vi "configuration UI.vi"() -> ()   [LabVIEW 2013, in "Shared Library Module editor node.lvclass"]
doc: "Platypus Framework 1.0.1.60\nNI Systems Engineering - National Instruments"
uses:
  Shared Library Module editor node.lvclass
  <vilib>/CEF_TreeControl/Node/NodeRef.ctl
  <vilib>/CEF_TreeControl/Node/NISE_CEF_Node.lvclass
  <vilib>/NI/AMC/Message Queue.ctl
  <vilib>/NI/AMC/Message.ctl
  <vilib>/NI/Tools/Keyed Array/KeyedArray.ctl
  <vilib>/CEF_TreeControl/Node/UserEventRef.ctl
  <vilib>/CEF_TreeControl/Controls/EventCluster.ctl
  <vilib>/TBM Modules/CLFN/configuration/Shared Library Module configuration.lvclass
  <vilib>/NI/Module Execution Interface/Engine Configuration/engine configuration.lvclass
  <vilib>/NI/Tag Bus Data Framework/Configuration Editor/Classes/Engine Parent/Engine Parent Editor Node.lvclass
  <vilib>/NI/Tag Bus Module Framework/root configuration/TBM configuration.lvclass/TBM configuration.ctl
  <vilib>/NI/Tag Bus/tag/tag descriptor.lvclass/tag descriptor.ctl
  <vilib>/TBM Modules/CLFN/configuration/Shared Library Module configuration.lvclass/Shared Library Module configuration.ctl
  <vilib>/NI/Tag Bus/tag/write tag name.vi
  <vilib>/TBM Modules/CLFN/configuration/Write args.vi
  <vilib>/TBM Modules/CLFN/configuration/Write dllpath.vi
  <vilib>/NI/Tag Bus Module Framework/root configuration/Read instance name.vi
  <vilib>/NI/Tag Bus Data Framework/Configuration Editor/Classes/Module editor node/Read Module Configuration.vi
  <vilib>/NI/Tag Bus Module Framework/root configuration/create GUID.vi
  <vilib>/NI/Tag Bus Module Framework/root configuration/TBM configuration.lvclass
  <vilib>/NI/Tag Bus Module Framework/module configuration/TBM module configuration.lvclass
  <vilib>/CEF_TreeControl/NISE_CEF_TreeControl.lvlib
  <vilib>/NI/Tag Bus Data Framework/Configuration Editor/Classes/Module editor node/module editor node.lvclass
  <vilib>/NI/Tag Bus Module Framework/channel/TBM channel.lvclass
  <vilib>/NI/Tools/Keyed Array/Tools_KeyedArray.lvlib
  <vilib>/NI/AMC/AMC.lvlib
panel:
  in  "Tab Control":T1(tab)
  in  "Remove Button":bool
  in  "Add Button":bool
  in  "channel":i32(listbox)
  in  "settings":bool
  in  "Open Button":bool
  in  "Library Path":path
  in  "Additional Arguments":string[](array[string])
  in  "user event":T2
  in  "main queue":T3
  in  "node ref":T4
  # "It is recommended that libraries are placed in the default search path. For example, on Linux RT this would be /usr/lib, while VxWorks places it at /ni-rt/system.\n\nIf this is the case, libraries can be referenced by name. To make the name cross-platform, wildcards can be specified.\n\nLibname.* becomes libname.dll on windows and libname.so on Linux.\n\nLibname*.* becomes Libname32.* on 32-bit operating systems/environments and Libname64.* on 64-bit operating systems/environments."
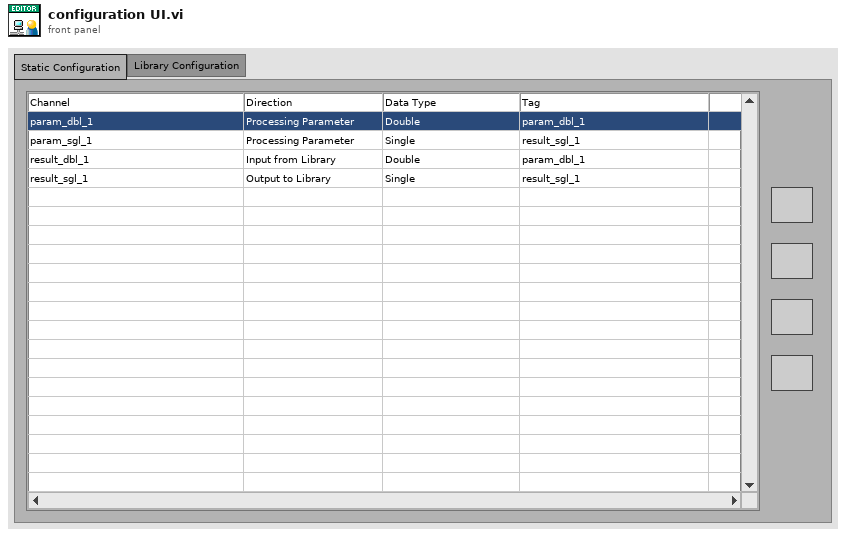
[diagram p1: front panel]
types:
  T1 = enum32{"Static Configuration", "Library Configuration"}
  T2 = typedef "NISE_CEF_Node.lvclass/UserEventRef.ctl" = refnum<user-event>
  T3 = typedef "AMC.lvlib/Message Queue.ctl" = refnum<queue>
  T4 = typedef "NISE_CEF_Node.lvclass/NodeRef.ctl" = refnum<data-value>
  T5 = typedef "NISE_CEF_TreeControl.lvlib/EventCluster.ctl" = cluster{"command":string, "data":string}
  T6 = typedef "Shared Library Module editor node.lvclass/table line.ctl" = cluster{"channel in":refnum<class "TBM channel.lvclass">, "tag name":string}
  T7 = typedef "TBM channel.lvclass/channel classification.ctl" = enum16{"input data", "output data", "processing parameter", "processing result"}
  T8 = typedef "tag bus.lvlib/tag descriptor.lvclass/Data Type.ctl" = enum16{"Double", "Single", "I64", "I32", "I16", "I8", "U64", "U32", "U16", "U8", "Boolean", "String", "Array of Double", "Array of Single", "Array of I64", "Array of I32", "Array of I16", "Array of I8", "Array of U64", "Array of U32", "Array of U16", "Array of U8", "Array of Boolean", "Array of String"}
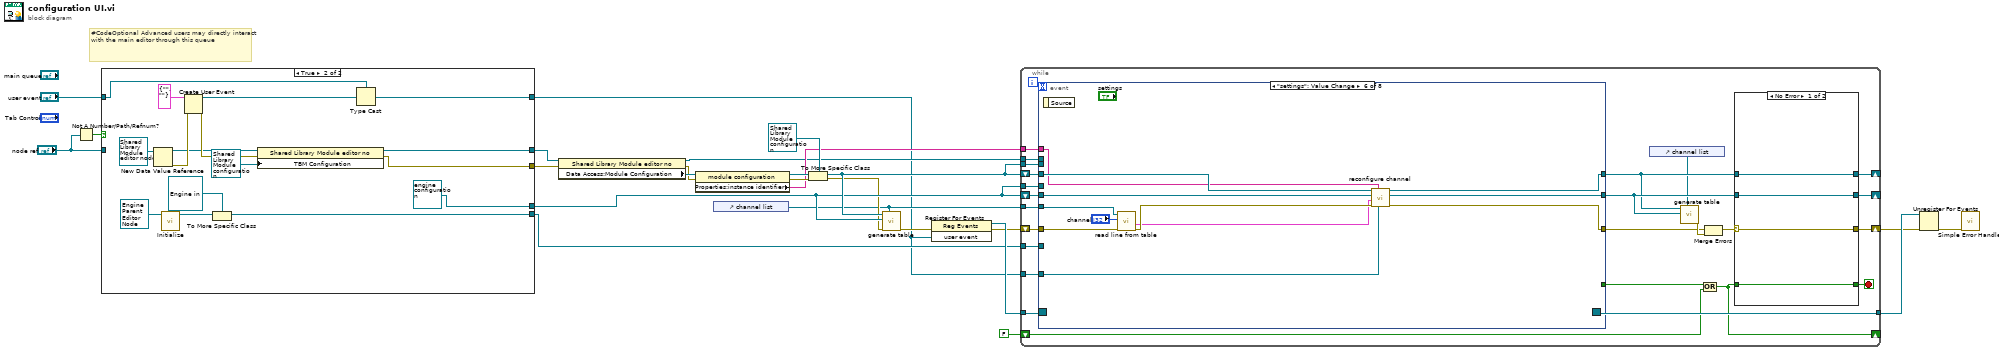
[diagram p0: block diagram]
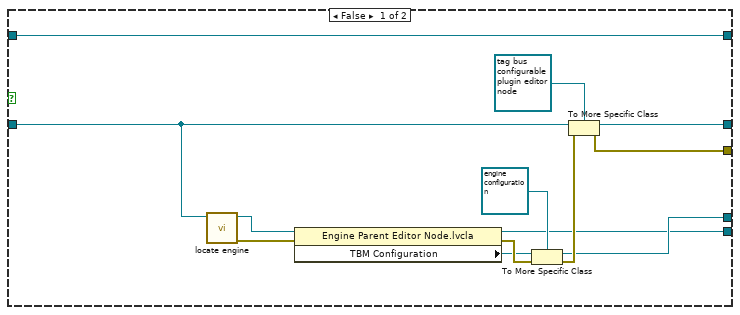
[diagram p2: hidden frame]
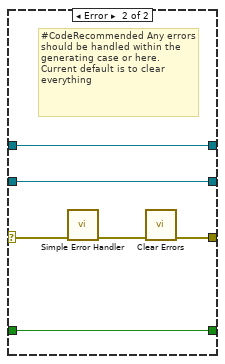
[diagram p3: hidden frame]
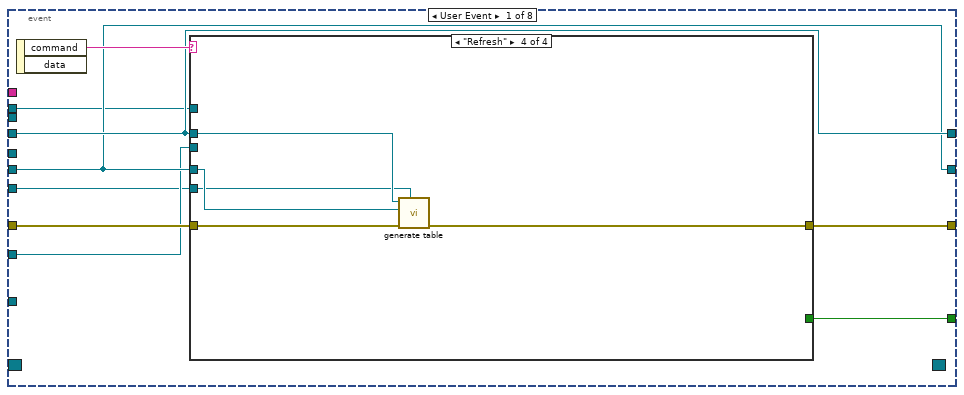
[diagram p4: hidden frame]
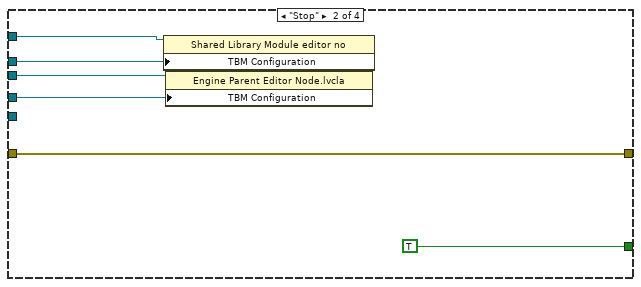
[diagram p6: hidden frame]
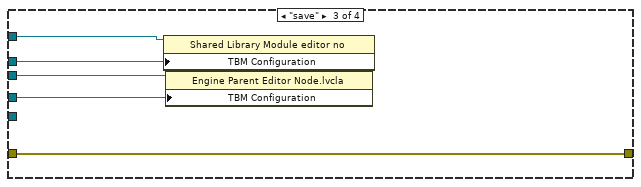
[diagram p7: hidden frame]
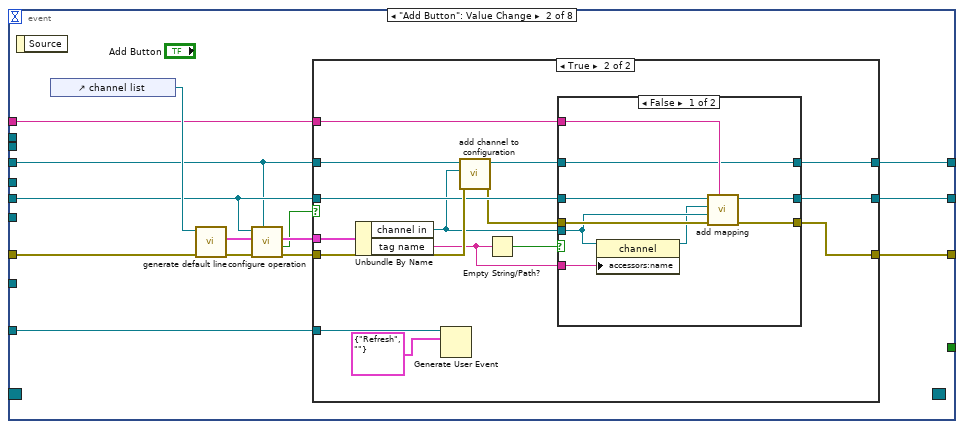
[diagram p8: hidden frame]
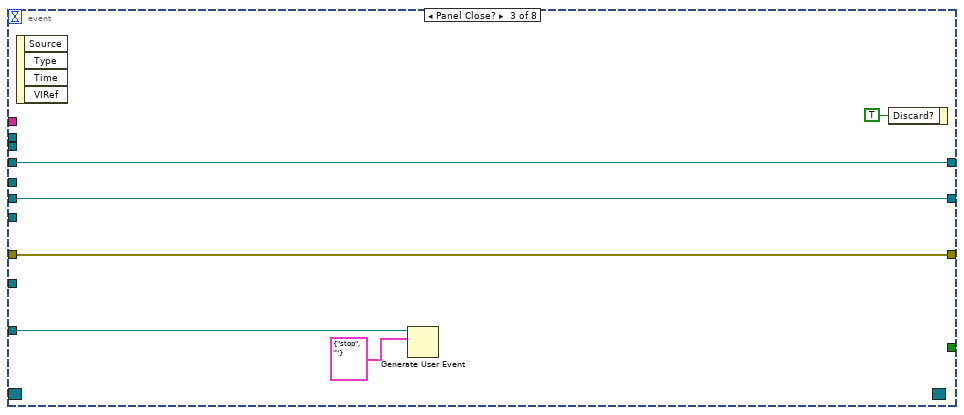
[diagram p11: hidden frame]
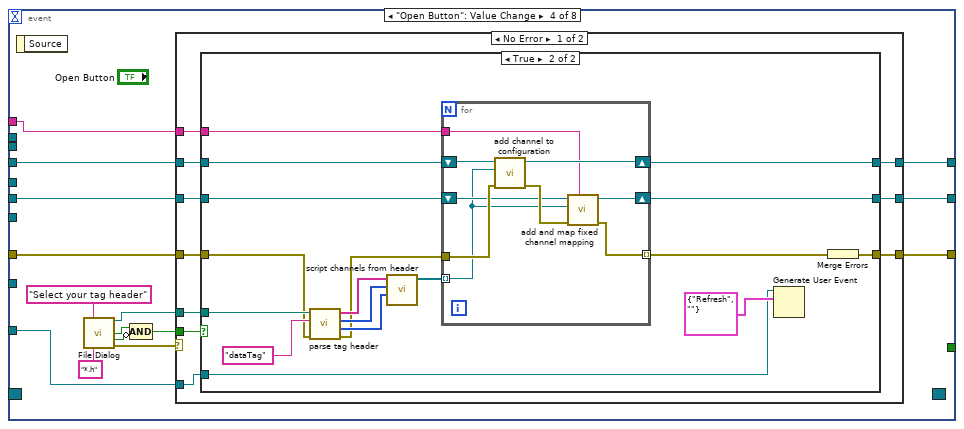
[diagram p12: hidden frame]
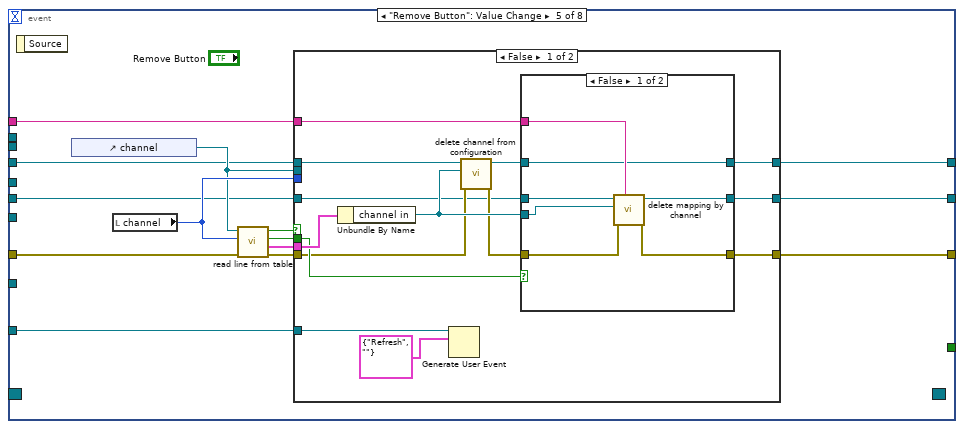
[diagram p15: hidden frame]
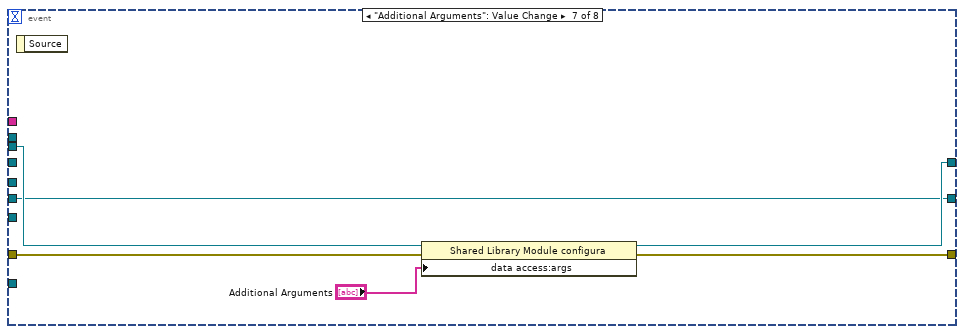
[diagram p18: hidden frame]
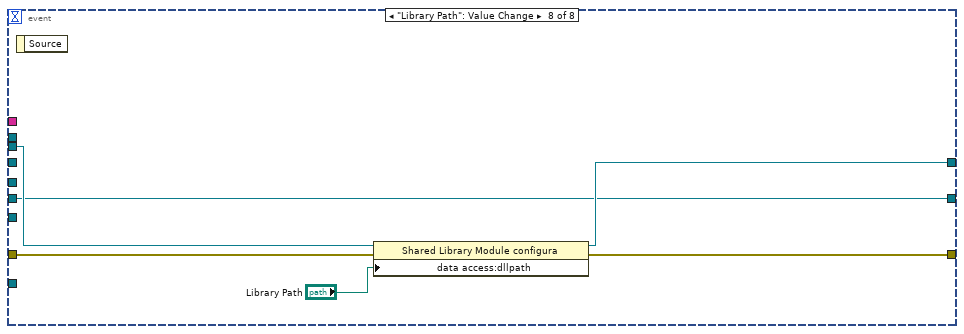
[diagram p19: hidden frame]
diagram:
  # "#CodeOptional Advanced users may directly interact with the main editor through this queue"
  n1 = Not A Number/Path/Refnum?(number/path/refnum="node ref") -> (NaN/Path/Refnum?=w16:bool)
  n2 = case shown="True" w16 {
    tunnel: "user event" -> [w38 w40]
    tunnel: [w38 w41] -> w1
    tunnel: "node ref" -> [w36 _]
    tunnel: [w35 w48] -> w8
    tunnel: [w34 w42] -> w14
    tunnel: [w27 refnum<class "engine configuration.lvclass"> refnum ("Engine Configuration")] -> w10
    tunnel: [w26 w45] -> w4
    frame False {
      n3 = call <vilib>:"locate engine.vi"("component"=w36) -> ("error out"=w31:errorcluster, "engine"=w33:refnum<data-value>)  [unwired: 9 in]
      n4 = property class="Engine Parent Editor Node.lvcla"(reference=w33, error in=w31) -> (reference out=w26:refnum<data-value>, error out=w30:errorcluster, "TBM Configuration"=w29:refnum<class "TBM configuration.lvclass">)
      n5 = To More Specific Class(target class=refnum<class "engine configuration.lvclass"> refnum ("engine configuration.lvclass"), reference=w29, error in=w30) -> (specific class reference=w27:refnum<class "engine configuration.lvclass">, error out=w28:errorcluster)
      n6 = To More Specific Class(target class=refnum<data-value> refnum ("data value reference"), reference=w36, error in=w28) -> (specific class reference=w35:refnum<data-value>, error out=w34:errorcluster)
    }
    frame True {
      n7 = New Data Value Reference(data value=refnum<class "Shared Library Module editor node.lvclass"> refnum ("tag bus configurable plugin editor node")) -> (data value reference=w47:refnum<data-value>, error out=w50:errorcluster)  [unwired: 1 in]
      n8 = call-dynamic "Initialize.vi"("Engine in"=refnum<class "Engine Parent Editor Node.lvclass"> refnum) -> ("data value reference"=w46:T4)  [unwired: 8 in, 2 out]
      n9 = Create User Event(user event datatype=T5 {"command"="", "data"=""} ("event data"), error in=w50) -> (user event=w53:refnum<user-event>, error out=w49:errorcluster)
      n10 = To More Specific Class(target class=refnum<data-value> refnum ("data value reference"), reference=w46) -> (specific class reference=w45:refnum<data-value>)  [unwired: 1 in, 1 out]
      n11 = property class="Shared Library Module editor no"(reference=w47, error in=w49, "TBM Configuration"=refnum<class "Shared Library Module configuration.lvclass"> refnum ("tag bus configurable plugin module configuration")) -> (reference out=w48:refnum<data-value>, error out=w42:errorcluster)
      n12 = Type Cast(type=w40, x=w53) -> (*(type *) &x=w41:T2)
    }
  }
  n13 = property class="Shared Library Module editor no"(reference=w8, error in=w14) -> (reference out=w3:refnum<data-value>, error out=w19:errorcluster, "Data Access:Module Configuration"=w20:refnum<class "TBM module configuration.lvclass">)
  n14 = property class="module configuration"(reference=w20, error in=w19) -> (reference out=w17:refnum<class "TBM module configuration.lvclass">, error out=w18:errorcluster, "Properties:instance identifier"=w13:string)
  n15 = control-ref of="channel list"() -> (w2:refnum<vi>)
  n16 = To More Specific Class(target class=refnum<class "Shared Library Module configuration.lvclass"> refnum ("tag bus configurable plugin module configuration"), reference=w17, error in=w18) -> (specific class reference=w11:refnum<class "Shared Library Module configuration.lvclass">, error out=w9:errorcluster)
  n17 = call "generate table.vi"("table"=w2, "error in"=w9, "engine configuration in"=w10, "Shared Library Module configuration in"=w11) -> ("error out"=w7:errorcluster)  [unwired: 7 in]
  n18 = register-events(error in=w7, w1) -> (reference out=w25:refnum<event-registration>, error out=w6:errorcluster)  [unwired: 1 in]
  n19 = while {
    tunnel: w25 -> [w79]
    tunnel: [w78] -> w24
    shift-right: [w72] -> w23
    shift-left: w6 -> [w77]
    shift-right: [w74] -> _
    shift-left: FALSE -> [w73]
    tunnel: w11 -> [w70]
    shift-right: [w66] -> _
    shift-left: w11 -> [w71]
    shift-right: [w67] -> _
    shift-left: w10 -> [w68]
    tunnel: w10 -> [w69]
    tunnel: w13 -> [w65]
    tunnel: w4 -> [w58]
    tunnel: w3 -> [w57]
    tunnel: w2 -> [w56]
    tunnel: w1 -> [w55]
    stop <- w76 stop-if-true
    n20 = event shown="[5] \"settings\": Value Change" {
      selector: w79 -> [_ _ _ _ _ _ _ _]
      dyn-events: [_ _ _ _ _ _ _ _] -> w78
      timeout: _ -> [_ _ _ _ _ _ _ _]
      tunnel: [w98 _ _ _ _ _ _ _] -> w75
      tunnel: [w96 w129 w165 w174 w236 w274 w280 w286] -> w60
      tunnel: w77 -> [w95 w128 w165 w173 w235 w275 w281 w287]
      tunnel: w71 -> [w94 w117 w163 w170 w231 w270 _ _]
      tunnel: w70 -> [_ _ _ _ _ _ w279 w285]
      tunnel: w69 -> [_ _ _ _ _ _ _ _]
      tunnel: w68 -> [w93 w118 w162 w171 w230 w271 w276 w282]
      tunnel: [w93 w122 w162 w172 w225 w268 w276 w282] -> w64
      tunnel: [w94 w121 w163 w169 w224 w269 w278 w284] -> w63
      tunnel: w65 -> [_ w120 _ w167 w226 w266 _ _]
      tunnel: w58 -> [w92 _ _ _ _ _ _ _]
      tunnel: w57 -> [w91 _ _ _ _ _ _ _]
      tunnel: w56 -> [w90 _ _ _ _ w267 _ _]
      tunnel: w55 -> [_ w116 w161 w166 w223 w264 _ _]
      event User Event {
        n21 = event-data() -> ("command"=w97:string)  [unwired: 1 in, 1 out]
        n22 = case shown="\"Refresh\"" w97 {
          tunnel: [_ TRUE _ _] -> w98
          tunnel: [w99 w104 w110 w112] -> w96
          tunnel: w95 -> [w99 w104 w110 w115]
          tunnel: w94 -> [_ w103 w109 w114]
          tunnel: w93 -> [_ w102 w108 w113]
          tunnel: w92 -> [_ w101 w107 _]
          tunnel: w91 -> [_ w100 w106 _]
          tunnel: w90 -> [_ _ _ w111]
          frame Default {
          }
          frame "Stop" {
            n23 = property class="Shared Library Module editor no"(reference=w100, "TBM Configuration"=w103) -> ()  [unwired: 1 in, 2 out]
            n24 = property class="Engine Parent Editor Node.lvcla"(reference=w101, "TBM Configuration"=w102) -> ()  [unwired: 1 in, 2 out]
          }
          frame "save" {
            n25 = property class="Shared Library Module editor no"(reference=w106, "TBM Configuration"=w109) -> ()  [unwired: 1 in, 2 out]
            n26 = property class="Engine Parent Editor Node.lvcla"(reference=w107, "TBM Configuration"=w108) -> ()  [unwired: 1 in, 2 out]
          }
          frame "Refresh" {
            n27 = call "generate table.vi"("table"=w111, "error in"=w115, "engine configuration in"=w113, "Shared Library Module configuration in"=w114) -> ("error out"=w112:errorcluster)  [unwired: 7 in]
          }
        }
      }
      event "Add Button": Value Change {
        n28 = event-data() -> ()  [unwired: 1 in, 1 out]
        n29 = control-ref of="channel list"() -> (w127:refnum<vi>)
        n30 = call "generate default line.vi"("error in"=w128, "operations table"=w127) -> ("error out"=w125:errorcluster, "line"=w126:T6)  [unwired: 8 in]
        n31 = call "configure operation.vi"("Shared Library Module configuration in"=w117, "error in"=w125, "line item in"=w126, "engine configuration in"=w118) -> ("error out"=w123:errorcluster, "success"=w119:bool, "line item out"=w124:T6)  [unwired: 4 in, 1 out]
        n32 = case shown="True" w119 {
          tunnel: [w132 w135] -> w129
          tunnel: w123 -> [w132 w145]
          tunnel: w118 -> [w131 w143]
          tunnel: w124 -> [_ w146]
          tunnel: w117 -> [w130 w147]
          tunnel: [w131 w142] -> w122
          tunnel: [w130 w136] -> w121
          tunnel: w120 -> [_ w139]
          tunnel: w116 -> [_ w133]
          frame False {
          }
          frame True {
            n33 = Unbundle By Name(w146) -> ("channel in"=w140:refnum<class "TBM channel.lvclass">, "tag name"=w138:string)
            n34 = Generate User Event(user event=w133, event data cluster=T5 {"command"="Refresh", "data"=""} ("event data")) -> ()  [unwired: 2 in, 2 out]
            n35 = call <vilib>:"add channel to configuration.vi"("error in"=w145, "TBM channel in"=w140, "Shared Library Module configuration in"=w147) -> ("error out"=w141:errorcluster, "Shared Library Module configuration out"=w137:refnum<class "Shared Library Module configuration.lvclass">)  [unwired: 7 in]
            n36 = Empty String/Path?(string/path=w138) -> (empty?=w144:bool)
            n37 = case shown="False" w144 {
              tunnel: w143 -> [w156 w159]
              tunnel: [w155 w159] -> w142
              tunnel: w141 -> [w154 w158]
              tunnel: w140 -> [w152 _]
              tunnel: w139 -> [w153 _]
              tunnel: w138 -> [w151 _]
              tunnel: [w149 w158] -> w135
              tunnel: w137 -> [w148 w157]
              tunnel: [w148 w157] -> w136
              frame False {
                n38 = property class="channel"(reference=w152, "accessors:name"=w151) -> (reference out=w150:refnum<class "TBM channel.lvclass">)  [unwired: 1 in, 1 out]
                n39 = call <vilib>:"add mapping.vi"("owner ID"=w153, "error in"=w154, "channel"=w152, "tag descriptor"=w150, "engine configuration"=w156) -> ("error out"=w149:errorcluster, "engine configuration out"=w155:refnum<class "engine configuration.lvclass">)  [unwired: 5 in]
              }
              frame True {
              }
            }
          }
        }
      }
      event Panel Close? {
        n40 = event-data() -> ()  [unwired: 1 in, 4 out]
        n41 = Generate User Event(user event=w161, event data cluster=T5 {"command"="stop", "data"=""} ("event data")) -> ()  [unwired: 2 in, 2 out]
        n42 = event-data("Discard?"=TRUE) -> ()  [unwired: 1 in, 1 out]
      }
      event "Open Button": Value Change {
        n43 = event-data() -> ()  [unwired: 1 in, 1 out]
        n44 = call "File Dialog"("prompt"="Select your tag header", "pattern (all files)"="*.h") -> ("selected path"=w168:path, "exists"=w177:bool, "cancelled"=w176:bool, "error out"=w178:errorcluster)  [unwired: 10 in]
        n45 = Compound Arithmetic op=AND(w177, invert w176) -> (w175:bool)
        n46 = case shown="No Error" w178 {
          tunnel: w175 -> [w190 _]
          tunnel: [w189 w222] -> w174
          tunnel: w173 -> [w188 w222]
          tunnel: [w186 w221] -> w172
          tunnel: w171 -> [w187 w221]
          tunnel: w170 -> [w184 w220]
          tunnel: [w185 w220] -> w169
          tunnel: w168 -> [w183 _]
          tunnel: w167 -> [w182 _]
          tunnel: w166 -> [w181 _]
          frame No Error {
            n47 = case shown="True" w190 {
              tunnel: [w193 w199] -> w189
              tunnel: w188 -> [w193 w205]
              tunnel: w187 -> [w192 w203]
              tunnel: [w192 w202] -> w186
              tunnel: [w191 w201] -> w185
              tunnel: w184 -> [w191 w204]
              tunnel: w183 -> [_ w206]
              tunnel: w182 -> [_ w196]
              tunnel: w181 -> [_ w194]
              frame False {
              }
              frame True {
                n48 = call <vilib>:"parse tag header.vi"("error in"=w205, "tag type name"="dataTag", "Path"=w206) -> ("error out"=w200:errorcluster, "classifications"=w210:T7[], "types"=w209:T8[], "names"=w208:string[])  [unwired: 5 in]
                n49 = call <vilib>:"script channels from header.vi"("classifications"=w210, "types"=w209, "names"=w208) -> ("channels"=w198:refnum<class "TBM channel.lvclass">[])  [unwired: 8 in]
                n50 = for {
                  shift-right: [w212] -> w201
                  shift-left: w204 -> [w219]
                  shift-right: [w213] -> w202
                  shift-left: w203 -> [w215]
                  tunnel: w200 -> [w218]
                  tunnel: w198 -> [w214] mode=indexing
                  tunnel: [w216] -> w197 mode=indexing
                  tunnel: w196 -> [w211]
                  n51 = call <vilib>:"add channel to configuration.vi"("error in"=w218, "TBM channel in"=w214, "Shared Library Module configuration in"=w219) -> ("error out"=w217:errorcluster, "Shared Library Module configuration out"=w212:refnum<class "Shared Library Module configuration.lvclass">)  [unwired: 7 in]
                  n52 = call <vilib>:"add and map fixed channel mapping.vi"("module instance"=w211, "error in"=w217, "fixed channel"=w214, "engine configuration in"=w215) -> ("error out"=w216:errorcluster, "engine configuration out"=w213:refnum<class "engine configuration.lvclass">)  [unwired: 6 in]
                }
                n53 = Generate User Event(user event=w194, event data cluster=T5 {"command"="Refresh", "data"=""} ("event data")) -> ()  [unwired: 2 in, 2 out]
                n54 = Merge Errors(w197) -> (w199:errorcluster)
              }
            }
          }
          frame Error {
          }
        }
      }
      event "Remove Button": Value Change {
        n55 = event-data() -> ()  [unwired: 1 in, 1 out]
        n56 = control-ref of="channel"() -> (w233:refnum<vi>)
        n57 = local read "channel"() -> (w234:i32)
        n58 = call "read line from table.vi"("error in"=w235, "line number"=w234, "operations table"=w233) -> ("error out"=w227:errorcluster, "line"=w232:T6, "empty tag?"=w228:bool, "empty channel?"=w229:bool)  [unwired: 5 in]
        n59 = case shown="False" w229 {
          tunnel: [w239 w262] -> w236
          tunnel: w234 -> [_ _]
          tunnel: w233 -> [_ _]
          tunnel: w232 -> [w250 _]
          tunnel: w231 -> [w248 w261]
          tunnel: w230 -> [w243 w263]
          tunnel: w228 -> [w249 _]
          tunnel: w227 -> [w246 w262]
          tunnel: w226 -> [w242 _]
          tunnel: [w241 w263] -> w225
          tunnel: [w240 w261] -> w224
          tunnel: w223 -> [w237 _]
          frame False {
            n60 = Unbundle By Name(w250) -> ("channel in"=w247:refnum<class "TBM channel.lvclass">)
            n61 = Generate User Event(user event=w237, event data cluster=T5 {"command"="Refresh", "data"=""} ("event data")) -> ()  [unwired: 2 in, 2 out]
            n62 = call <vilib>:"delete channel from configuration.vi"("error in"=w246, "TBM channel in"=w247, "Shared Library Module configuration in"=w248) -> ("error out"=w244:errorcluster, "Shared Library Module configuration out"=w245:refnum<class "Shared Library Module configuration.lvclass">)  [unwired: 7 in]
            n63 = case shown="False" w249 {
              tunnel: w247 -> [w256 _]
              tunnel: w245 -> [w251 w258]
              tunnel: w244 -> [w254 w259]
              tunnel: w243 -> [w257 w260]
              tunnel: w242 -> [w255 _]
              tunnel: [w253 w260] -> w241
              tunnel: [w252 w259] -> w239
              tunnel: [w251 w258] -> w240
              frame False {
                n64 = call <vilib>:"delete mapping by channel.vi"("owner ID"=w255, "error in"=w254, "channel"=w256, "engine configuration in"=w257) -> ("error out"=w252:errorcluster, "engine configuration out"=w253:refnum<class "engine configuration.lvclass">)  [unwired: 6 in]
              }
              frame True {
              }
            }
          }
          frame True {
          }
        }
      }
      event "settings": Value Change {
        n65 = event-data() -> ()  [unwired: 1 in, 1 out]
        n66 = call "read line from table.vi"("error in"=w275, "line number"="channel", "operations table"=w267) -> ("error out"=w273:errorcluster, "line"=w265:T6)  [unwired: 5 in, 2 out]
        n67 = call "reconfigure channel.vi"("user event"=w264, "instance identifier"=w266, "error in"=w273, "line"=w265, "Data Access:Engine Configuration"=w271, "Shared Library Module configuration in"=w270) -> ("error out"=w274:errorcluster, "engine configuration out"=w268:refnum<class "engine configuration.lvclass">, "Shared Library Module configuration out"=w269:refnum<class "Shared Library Module configuration.lvclass">)  [unwired: 3 in]
      }
      event "Additional Arguments": Value Change {
        n68 = event-data() -> ()  [unwired: 1 in, 1 out]
        n69 = property class="Shared Library Module configura"(reference=w279, error in=w281, "data access:args"="Additional Arguments") -> (reference out=w278:refnum<class "Shared Library Module configuration.lvclass">, error out=w280:errorcluster)
      }
      event "Library Path": Value Change {
        n70 = event-data() -> ()  [unwired: 1 in, 1 out]
        n71 = property class="Shared Library Module configura"(reference=w285, error in=w287, "data access:dllpath"="Library Path") -> (reference out=w284:refnum<class "Shared Library Module configuration.lvclass">, error out=w286:errorcluster)
      }
    }
    n72 = control-ref of="channel list"() -> (w62:refnum<vi>)
    n73 = call "generate table.vi"("table"=w62, "engine configuration in"=w64, "Shared Library Module configuration in"=w63) -> ("error out"=w61:errorcluster)  [unwired: 8 in]
    n74 = Or(x=w75, y=w73) -> (x .or. y?=w74:bool)
    n75 = Merge Errors(w60, w61) -> (w59:errorcluster)
    n76 = case shown="No Error" w59 {
      selector: w59 -> [w80 w88]
      tunnel: [w83 w89] -> w76
      tunnel: w74 -> [w83 w89]
      tunnel: [w80 w86] -> w72
      tunnel: w64 -> [w81 w85]
      tunnel: [w81 w85] -> w67
      tunnel: w63 -> [w82 w84]
      tunnel: [w82 w84] -> w66
      frame No Error {
      }
      frame Error {
        # "#CodeRecommended Any errors should be handled within the generating case or here. Current default is to clear everything"
        n77 = call <vilib>:"Simple Error Handler.vi"("error in (no error)"=w88) -> ("error out"=w87:errorcluster)  [unwired: 4 in, 4 out]
        n78 = call <vilib>:"Clear Errors.vi"("error in (no error)"=w87) -> ("error out"=w86:errorcluster)  [unwired: 6 in]
      }
    }
  }
  n79 = Unregister For Events(event registration refnum=w24, error in=w23) -> (error out=w5:errorcluster)
  n80 = call <vilib>:"Simple Error Handler.vi"("error in (no error)"=w5) -> ()  [unwired: 4 in, 5 out]
